vi "Set 2D Array Double Complex.vi"(5 "use temporary file? (F)":bool, 8 "error in":errorcluster, 9 "value":cdb[][](array[numeric]), 10 "variable name":string, 11 "GOLPI ref. in":T1={"pipe handle"={"lv_proc.dll file path"=path "", "process instance handle"=[], "debug mode"=FALSE, "debug data"=[]}, "fast read timeout [ms]"=500, "fast read settle time [ms]"=10, "fast read to multiple [ms]"=1, "max elements per input line"=100, "slow read timeout [ms]"=5000, "stdin double format specifier"="%_16e", "max elements per stdout output column"=100, "console mode bitstream"=FALSE, "bitstream first read timeout [ms]"=1000, "bitstream read timeout [ms]"=50, "struct transfer possible"=FALSE, "matlab mode"=FALSE, "var pipe write timeout [ms]"=5000, "variable pipe mode"=FALSE, "variable pipe buffer size [Bytes]"=10000000, "variable pipe block size [Bytes]"=1000000} {"variable pipe block size [Bytes]" format="%.0p"; "variable pipe buffer size [Bytes]" format="%.0p"}) -> (0 "error out":errorcluster, 3 "GOLPI ref. out":T1={"pipe handle"={"lv_proc.dll file path"=path "", "process instance handle"=[], "debug mode"=FALSE, "debug data"=[]}, "fast read timeout [ms]"=500, "fast read settle time [ms]"=10, "fast read to multiple [ms]"=1, "max elements per input line"=100, "slow read timeout [ms]"=5000, "stdin double format specifier"="%_16e", "max elements per stdout output column"=100, "console mode bitstream"=FALSE, "bitstream first read timeout [ms]"=1000, "bitstream read timeout [ms]"=50, "struct transfer possible"=FALSE, "matlab mode"=FALSE, "var pipe write timeout [ms]"=5000, "variable pipe mode"=FALSE, "variable pipe buffer size [Bytes]"=10000000, "variable pipe block size [Bytes]"=1000000} {"variable pipe block size [Bytes]" format="%.0p"; "variable pipe buffer size [Bytes]" format="%.0p"})   [LabVIEW 2020, in "GOLPI library.lvlib"]
doc: "Part of polymorph Set Variable.vi"
uses:
  GOLPI library.lvlib
  Public/GOLPI reference Type Def.ctl
  LV Process source distribution/Pipe Handle.ctl
  LV Process source distribution/LV Process library.lvlib
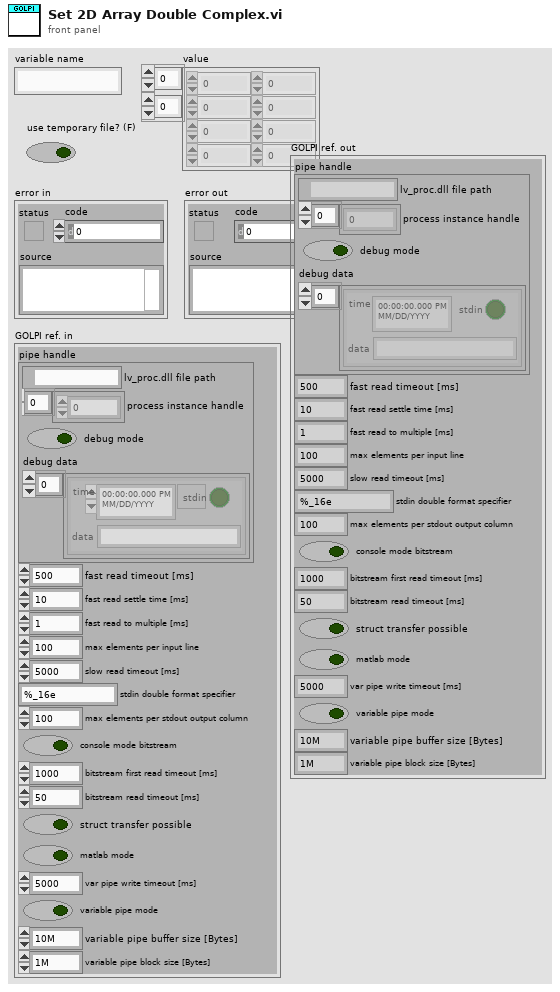
[diagram p1: front panel]
types:
  T1 = typedef "GOLPI library.lvlib/GOLPI reference Type Def.ctl" = cluster{"pipe handle":T2, "fast read timeout [ms]":u32, "fast read settle time [ms]":u32, "fast read to multiple [ms]":u32, "max elements per input line":u32, "slow read timeout [ms]":u32, "stdin double format specifier":string, "max elements per stdout output column":u32, "console mode bitstream":bool, "bitstream first read timeout [ms]":u32, "bitstream read timeout [ms]":u32, "struct transfer possible":bool, "matlab mode":bool, "var pipe write timeout [ms]":u32, "variable pipe mode":bool, "variable pipe buffer size [Bytes]":u32, "variable pipe block size [Bytes]":u32}
  T2 = typedef "LV Process library.lvlib/Pipe Handle.ctl" = cluster{"lv_proc.dll file path":path, "process instance handle":u32[], "debug mode":bool, "debug data":cluster{"time":timestamp, "stdin":bool, "data":string}[]}
  T3 = typedef "GOLPI library.lvlib/Transfer Mode.ctl" = enum16{"Matlab", "stdio", "temp file", "bitstream", "pipe"}
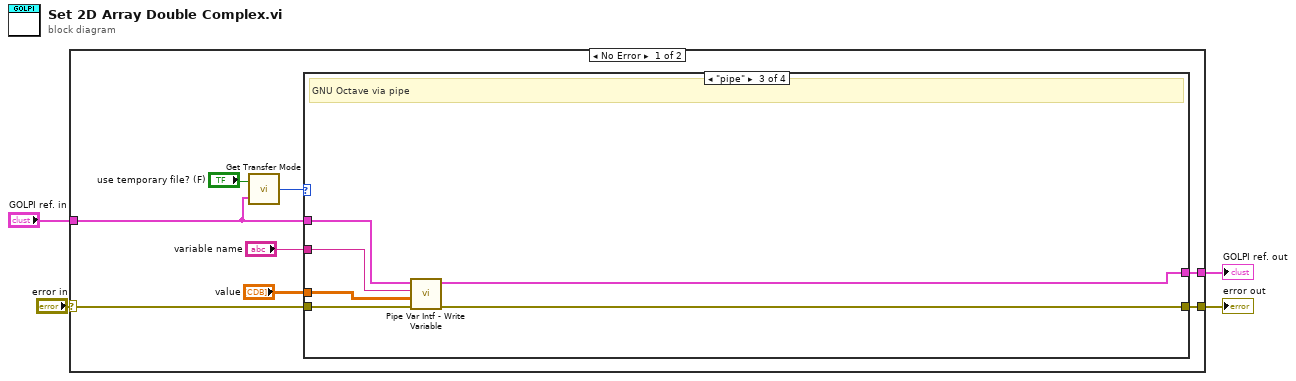
[diagram p0: block diagram]
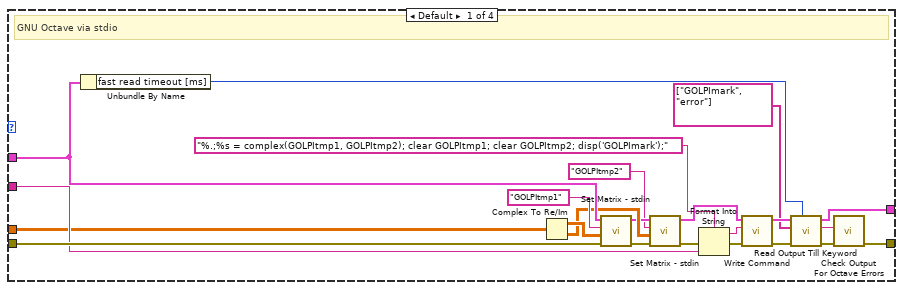
[diagram p2: hidden frame]
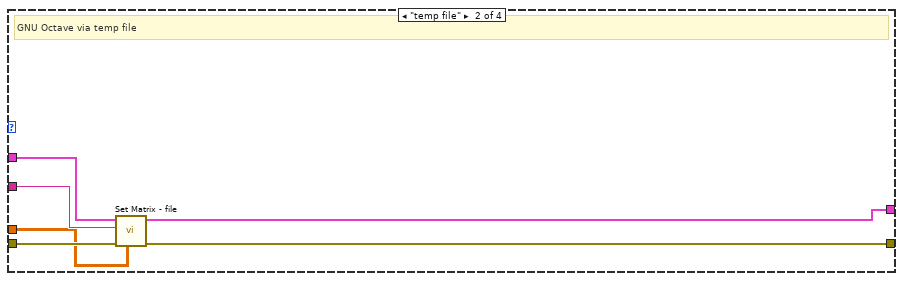
[diagram p3: hidden frame]
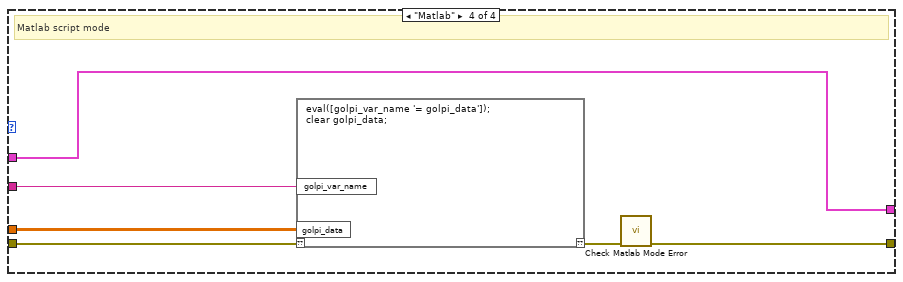
[diagram p4: hidden frame]
diagram:
  n1 = case shown="No Error" "error in" {
    selector: "error in" -> [w12 w55]
    tunnel: [w10 w55] -> w4
    tunnel: "GOLPI ref. in" -> [w6 w54]
    tunnel: [w11 w54] -> w1
    frame No Error {
      n2 = call "Get Transfer Mode.vi"("GOLPI ref."=w6, "use temporary file? (F)"="use temporary file? (F)") -> ("mode"=w7:T3)
      n3 = case shown="\"pipe\"" w7 {
        tunnel: w12 -> [w35 w41 w47 w53]
        tunnel: [w34 w40 w46 w50] -> w11
        tunnel: [w33 w39 w45 w48] -> w10
        tunnel: "variable name" -> [w32 w38 w44 w51]
        tunnel: w6 -> [w31 w37 w43 w50]
        tunnel: "value" -> [w30 w36 w42 w52]
        frame Default {
          # "GNU Octave via stdio"
          n4 = Unbundle By Name(w31) -> ("fast read timeout [ms]"=w13:u32)
          n5 = Complex To Re/Im(x + iy=w30) -> (x=w29:dbl[][], y=w27:dbl[][])
          n6 = call "Set Matrix - stdin.vi"("error in"=w35, "value"=w29, "variable name"="GOLPItmp1", "GOLPI ref. in"=w31) -> ("error out"=w25:errorcluster, "GOLPI ref. out"=w26:T1)  [unwired: 6 in]
          n7 = call "Set Matrix - stdin.vi"("error in"=w25, "value"=w27, "variable name"="GOLPItmp2", "GOLPI ref. in"=w26) -> ("error out"=w17:errorcluster, "GOLPI ref. out"=w23:T1)  [unwired: 6 in]
          n8 = Format Into String(format string="%.;%s = complex(GOLPItmp1, GOLPItmp2); clear GOLPItmp1; clear GOLPItmp2; disp('GOLPImark');" ("command"), error in=w17, w32) -> (resulting string=w14:string, error out=w16:errorcluster)  [unwired: 1 in]
          n9 = call "Write Command.vi"("error in"=w16, "command"=w14, "GOLPI ref. in"=w23) -> ("error out"=w15:errorcluster, "GOLPI ref. out"=w22:T1)  [unwired: 7 in]
          n10 = call "Read Output Till Keyword.vi"("timeout [ms]"=w13, "error in"=w15, "keywords"=string[] ["GOLPImark", "error"], "GOLPI ref. in"=w22) -> ("error out"=w19:errorcluster, "read buffer"=w20:string, "GOLPI ref. out"=w34:T1)  [unwired: 4 in, 1 out]
          n11 = call "Check Output For Octave Errors.vi"("error in"=w19, "read buffer"=w20) -> ("error out"=w33:errorcluster)  [unwired: 9 in]
        }
        frame "temp file" {
          # "GNU Octave via temp file"
          n12 = call "Set Matrix - file.vi"("cmplx double array"=w36, "error in (no error)"=w41, "variable name"=w38, "GOLPI ref. in"=w37) -> ("error out"=w39:errorcluster, "GOLPI ref. out"=w40:T1)  [unwired: 6 in]
        }
        frame "pipe" {
          # "GNU Octave via pipe"
          n13 = call "Pipe Var Intf - Write Variable.vi"("error in (no error)"=w47, "data in"=w42, "variable name"=w44, "GOLPI ref. in"=w43) -> ("error out"=w45:errorcluster, "GOLPI ref. out"=w46:T1)  [unwired: 6 in]
        }
        frame "Matlab" {
          # "Matlab script mode"
          n14 = script code="eval([golpi_var_name '= golpi_data']);\nclear golpi_data;"("??"=w53, "golpi_var_name"=w51, "golpi_data"=w52) -> ("??"=w49:errorcluster)
          n15 = call "Check Matlab Mode Error.vi"("error in"=w49) -> ("error out"=w48:errorcluster)  [unwired: 10 in]
        }
      }
    }
    frame Error {
    }
  }
  "error out" <- w4
  "GOLPI ref. out" <- w1
